vi "Lift PID Control for tester.vi"(0 "Use Motion Profiler":bool, 1 "Limit Switches":T6, 5 "Operator Gamepad":T10, 7 "Lift Potentionmeter":T7, 9 "Lift Deadband":dbl=0.1, 11 "Gains UP":cluster{"P":dbl, "I":dbl, "D":dbl}={"P"=0.1, "I"=0.0, "D"=0.0}, 12 "Gains DOWN":cluster{"P":dbl, "I":dbl, "D":dbl}={"P"=0.1, "I"=0.0, "D"=0.0}, 13 "Limit":dbl=0.666, 14 "Time to Wait":i32=10) -> (4 "Motor output":dbl format="%#_13g", 10 "Tolerable?":bool)   [LabVIEW 2014]
uses:
  <vilib>/Rock Robotics/WPI/Joystick/WPI_JoystickDevRef.ctl
  <vilib>/Rock Robotics/WPI/Joystick/WPI_JoystickDeviceEnum.ctl
  <vilib>/Rock Robotics/WPI/Potentiometer/WPI_PotentiometerDevRef.ctl
  <vilib>/Rock Robotics/SystemInterfaces/Typedef/FPGA_TypedefAnalogModule.ctl
  <vilib>/Rock Robotics/SystemInterfaces/AI/FPGA_AIChannel.ctl
  <vilib>/Rock Robotics/WPI/Switch/WPI_SwitchDevRef.ctl
  <vilib>/Rock Robotics/SystemInterfaces/DIO/FPGA_DIOChannel.ctl
  <vilib>/Rock Robotics/SystemInterfaces/Typedef/FPGA_TypedefDigitalModule.ctl
  <vilib>/Rock Robotics/SystemInterfaces/Counter/FPGA_CounterCtrSystemIndex.ctl
  SubVI/Motion Profiler/Max profiles.ctl
  <vilib>/Rock Robotics/WPI/DriverStation/WPI_DriverStationRobotMode2.ctl
  Robot Global Data.vi
  <vilib>/Rock Robotics/Network Tables/SD Write Number.vi
panel:
  in  "Max profiles":T1={"Max jerk"=150.0, "Max acceleration"=15.0, "Max Velocity"=20.0}
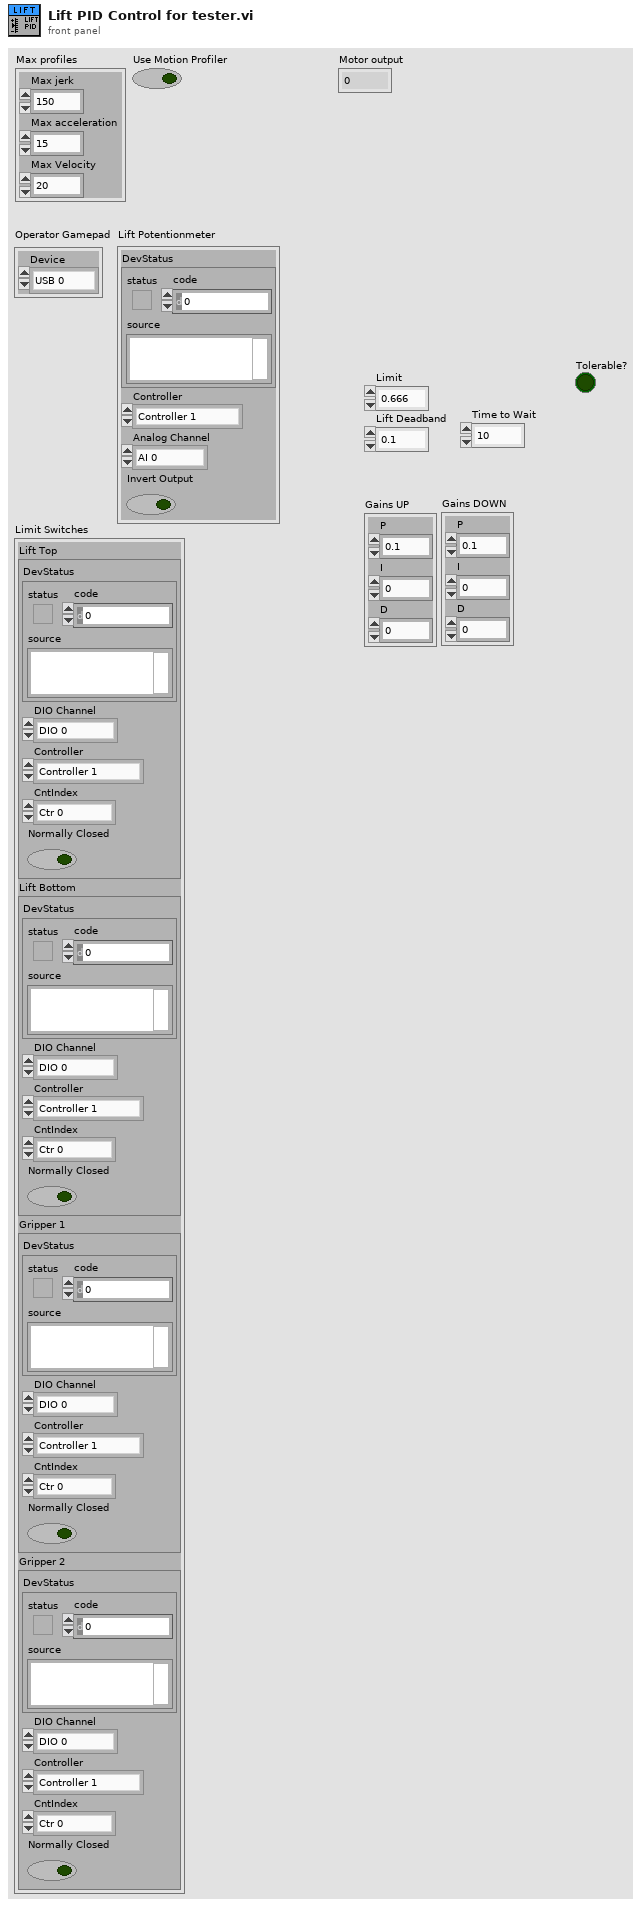
[diagram p1: front panel]
types:
  T1 = typedef "Max profiles.ctl" = cluster{"Max jerk":dbl, "Max acceleration":dbl, "Max Velocity":dbl}
  T2 = typedef "WPI_SwitchDevRef.ctl" = cluster{"DevStatus":errorcluster, "DIO Channel":T3, "Controller":T4, "CntIndex":T5, "Normally Closed":bool}
  T3 = typedef "FPGA_DIOChannel.ctl" = enum8{"DIO 0", "DIO 1", "DIO 2", "DIO 3", "DIO 4", "DIO 5", "DIO 6", "DIO 7", "DIO 8", "DIO 9", "DIO MXP 0", "DIO MXP 1", "DIO MXP 2", "DIO MXP 3", "DIO MXP 4", "DIO MXP 5", "DIO MXP 6", "DIO MXP 7", "DIO MXP 8", "DIO MXP 9", "DIO MXP 10", "DIO MXP 11", "DIO MXP 12", "DIO MXP 13", "DIO MXP 14", "DIO MXP 15", "Invalid"}
  T4 = typedef "FPGA_TypedefDigitalModule.ctl" = enum16{"Controller 1"}
  T5 = typedef "FPGA_CounterCtrSystemIndex.ctl" = enum8{"Ctr 0", "Ctr 1", "Ctr 2", "Ctr 3", "Ctr 4", "Ctr 5", "Ctr 6", "Ctr 7", "Invalid"}
  T6 = cluster{"Lift Top":T2, "Lift Bottom":T2, "Gripper 1":T2, "Gripper 2":T2}
  T7 = typedef "WPI_PotentiometerDevRef.ctl" = cluster{"DevStatus":errorcluster, "Controller":T8, "Analog Channel":T9, "Invert Output":bool}
  T8 = typedef "FPGA_TypedefAnalogModule.ctl" = enum16{"Controller 1"}
  T9 = typedef "FPGA_AIChannel.ctl" = enum8{"AI 0", "AI 1", "AI 2", "AI 3", "AI MXP 0", "AI MXP 1", "AI MXP 2", "AI MXP 3", "Invalid"}
  T10 = typedef "WPI_JoystickDevRef.ctl" = cluster{"Device":T11}
  T11 = typedef "WPI_JoystickDeviceEnum.ctl" = enum16{"USB 0", "USB 1", "USB 2", "USB 3", "USB 4", "USB 5"}
  T12 = typedef "WPI_DriverStationRobotMode2.ctl" = enum16{"Autonomous Disabled", "Autonomous Enabled", "Teleop Disabled", "Teleop Enabled", "Disconnected", "Finish", "Test Disabled", "Test Enabled", "Emergency Stopped"}
  T13 = typedef "Profiler Shift.ctl" = cluster{"TimeSegments":T14, "Current Setpoint":dbl, "Location at last setpoint change":dbl, "Time at last setpoint change":dbl, "Last Position setpoint":dbl, "Disable Profiler?":bool, "Time at last run":dbl, "Position at last call":dbl}
  T14 = typedef "TimeSegments.ctl" = cluster{"TimeSegments":T15[], "inital velocity":dbl, "inital acceleration":dbl}
  T15 = typedef "TimeSegment.ctl" = cluster{"StartTime":dbl, "TimePeriod":dbl, "PositionAtEnd":dbl, "VelocityAtEnd":dbl}
  T16 = cluster{"Error":dbl, "millisecond timer value":u32, "To Shift Register":dbl}
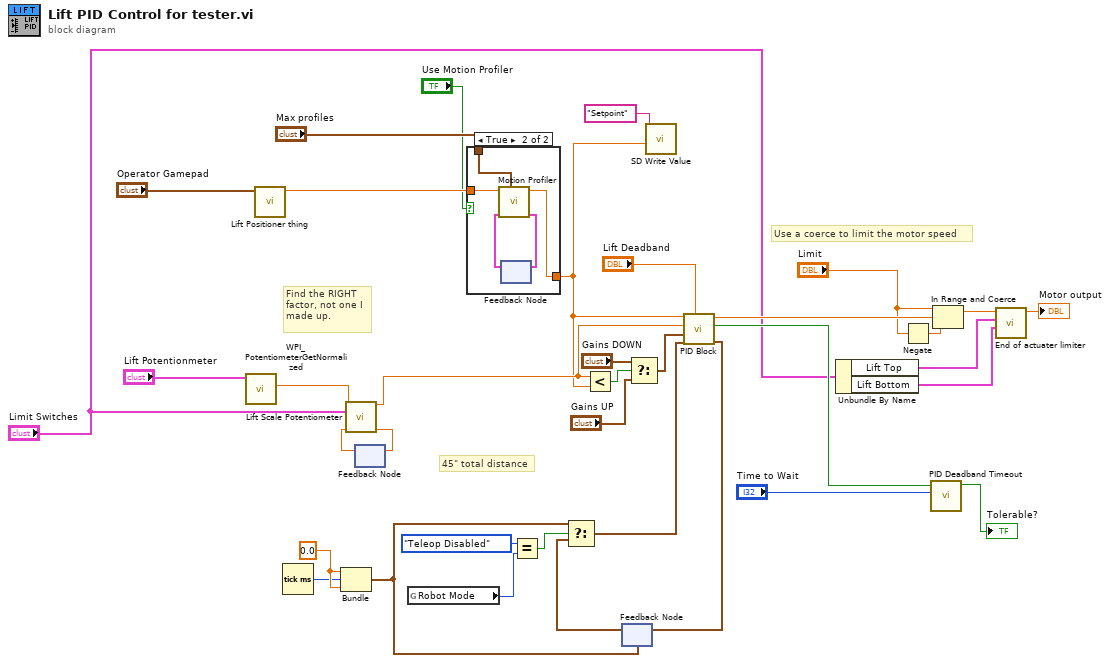
[diagram p0: block diagram]
diagram:
  w24 = 0.0
  # "45\" total distance"
  # "Find the RIGHT\nfactor, not one I\nmade up."
  # "Use a coerce to limit the motor speed"
  n1 = call <vilib>:"WPI_PotentiometerGetNormalized.vi"("PotDevRef"="Lift Potentionmeter") -> ("Normalized Value"=w6:dbl)  [unwired: 8 in, 2 out]
  n2 = call "Lift Positioner thing.vi"("Operator Gamepad"="Operator Gamepad") -> ("Setpoint"=w10:dbl)  [unwired: 10 in]
  n3 = Tick Count (ms)() -> (millisecond timer value=w23:u32)
  n4 = Bundle(w24, "millisecond timer value"=w23, w24) -> (w20:cluster{dbl, "millisecond timer value":u32, dbl})  [unwired: 1 in]
  n5 = feedback #1() -> (w5:dbl)  [unwired: 1 in]
  n6 = call "Lift Scale Potentiometer.vi"("Potentiometer In"=w6, "Limit Switches"="Limit Switches", "From Shift"=w5) -> ("Scaled Value Out"=w3:dbl, "To Shift"=w4:dbl)  [unwired: 11 in]
  n7 = feedback-in #1(w4) -> ()
  n8 = global read "Robot Global Data.vi" "Robot Mode"() -> (w17:T12)
  n9 = case shown="True" "Use Motion Profiler" {
    tunnel: w10 -> [w37 w42]
    tunnel: "Max profiles" -> [_ w41]
    tunnel: [w37 w38] -> w2
    frame False {
    }
    frame True {
      n10 = feedback #2() -> (w39:T13)  [unwired: 1 in]
      n11 = call "Motion Profiler.vi"("Max profiles"=w41, "From shift"=w39, "Setpoint"=w42) -> ("To Shift"=w40:T13, "Motion Profiler Setpoint output"=w38:dbl)  [unwired: 7 in]
      n12 = feedback-in #2(w40) -> ()
    }
  }
  n13 = Equal?(x=WPI_DriverStationRobotMode2."Teleop Disabled", y=w17) -> (x = y?=w19:bool)
  n14 = Less?(x=w3, y=w2) -> (x < y?=w12:bool)
  n15 = feedback #3(w20) -> (w21:cluster{dbl, "millisecond timer value":u32, dbl})
  n16 = Select(t=w20, s=w19, f=w21) -> (s? t:f=w22:cluster{dbl, "millisecond timer value":u32, dbl})
  n17 = Select(t="Gains DOWN", s=w12, f="Gains UP") -> (s? t:f=w15:cluster{"P":dbl, "I":dbl, "D":dbl})
  n18 = call-poly <vilib>:"SD Write Value.vi"("Numeric"=w2, "Name"="Setpoint") -> ()  [unwired: 8 in, 2 out]
  n19 = call "PID Block.vi"("Deadband"="Lift Deadband", "From Shift"=w22, "Gains"=w15, "Position"=w3, "Setpoint"=w2) -> ("To Shift"=w35:T16, "Tolerable?"=w34:bool, "Output"=w30:dbl)  [unwired: 4 in]
  n20 = feedback-in #3(w35) -> ()
  n21 = Unbundle By Name("Limit Switches") -> ("Lift Top"=w25:T2, "Lift Bottom"=w26:T2)
  n22 = Negate(x="Limit") -> (-x=w28:dbl)
  n23 = call "PID Deadband Timeout.vi"("Time to Wait"="Time to Wait", "In deadband range?"=w34) -> ("Deadband Timed-out"=→"Tolerable?":bool)  [unwired: 9 in]
  n24 = In Range and Coerce(upper limit="Limit", x=w30, lower limit=w28) -> (coerced(x)=w29:dbl)  [unwired: 1 out]
  n25 = call "End of actuater limiter.vi"("Lower limit switch"=w26, "Upper limit switch"=w25, "Motor input"=w29) -> ("Motor output"=→"Motor output":dbl)  [unwired: 8 in]
